vi "Write comments to sxp-file.vi"(5 "Location":enum16{"Beginning", "End"}(ring), 7 "Comment character":string="!", 8 "error in (no error)":errorcluster, 10 "Comment lines":string[](array[string]), 11 "file path":path) -> (0 "error out":errorcluster, 3 "file path out":path)   [LabVIEW 2020]
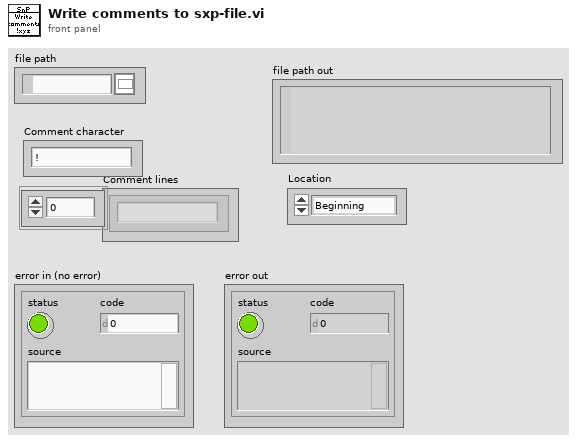
[diagram p1: front panel]
types:
  T1 = enum16{"open", "replace", "create", "open or create", "replace or create", "replace or create with confirmation"}
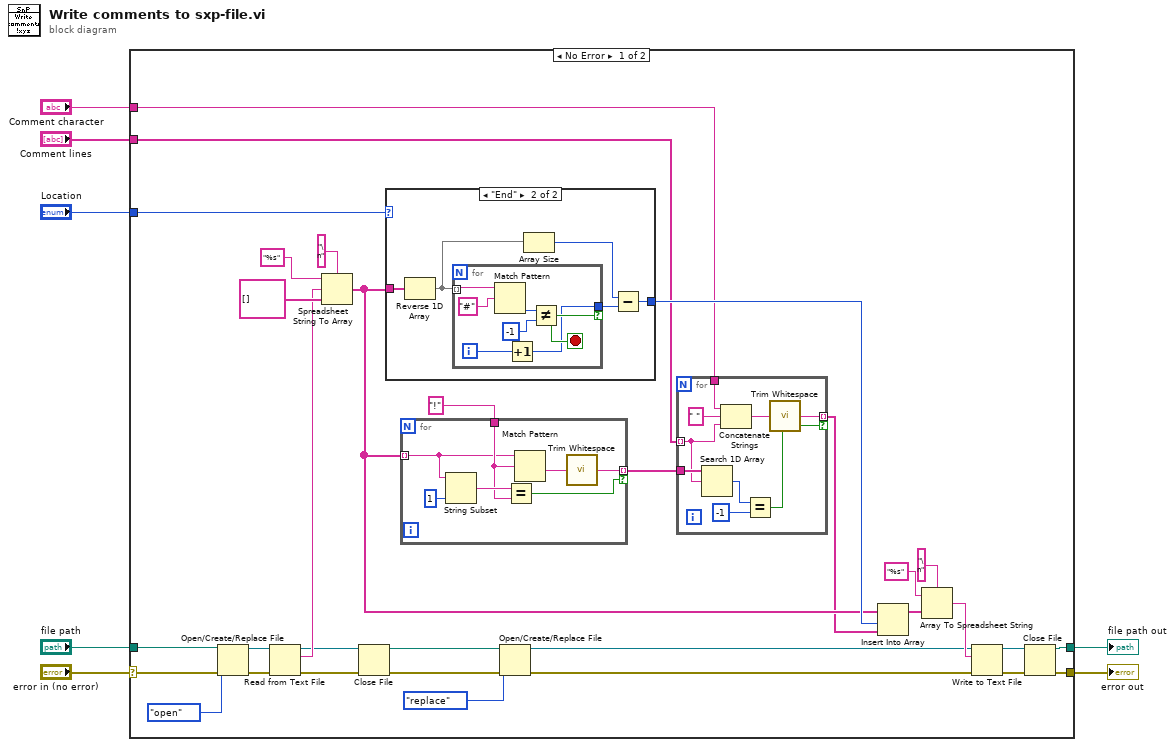
[diagram p0: block diagram]
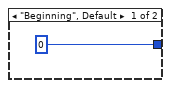
[diagram p2: hidden frame]
diagram:
  n1 = case shown="No Error" "error in (no error)" {
    selector: "error in (no error)" -> [w37 w70]
    tunnel: [w39 w70] -> w7
    tunnel: [w38 w69] -> w6
    tunnel: "Comment character" -> [w9 _]
    tunnel: "Comment lines" -> [w8 _]
    tunnel: "Location" -> [w24 _]
    tunnel: "file path" -> [w20 w69]
    frame No Error {
      n2 = Open/Create/Replace File(file path (use dialog)=w20, error in=w37, operation (0:open)=T1."open") -> (refnum out=w33:refnum<file>, error out=w32:errorcluster)  [unwired: 3 in, 1 out]
      n3 = Read from Text File(file (use dialog)=w33, error in=w32) -> (refnum out=w18:refnum<file>, text=w31:string, error out=w19:errorcluster)  [unwired: 2 in, 1 out]
      n4 = Spreadsheet String To Array(delimiter (Tab)="\n", format string="%s", spreadsheet string=w31, array type (2D Dbl)=string[] []) -> (array=w12:string[])
      n5 = Close File(refnum=w18, error in=w19) -> (path=w17:path, error out=w16:errorcluster)
      n6 = case shown="\"End\"" w24 {
        tunnel: [0 w57] -> w23
        tunnel: w12 -> [_ w58]
        frame "Beginning", Default {
        }
        frame "End" {
          n7 = Reverse 1D Array(array=w58) -> (reversed array=w59:string[])
          n8 = for {
            tunnel: w59 -> [w68] mode=indexing
            tunnel: [w62] -> w61 if=w64
            i -> [w63]
            stop <- w64 stop-if-true
            n9 = Match Pattern(string=w68, regular expression="#") -> (offset past match=w66:i32)  [unwired: 1 in, 3 out]
            n10 = Increment(x=w63) -> (x+1=w62:i32)
            n11 = Not Equal?(x=w66, y=-1) -> (x != y?=w64:bool)
          }
          n12 = Array Size(array=w59) -> (size(s)=w60:i32)
          n13 = Subtract(x=w60, y=w61) -> (x-y=w57:i32)
        }
      }
      n14 = for {
        tunnel: w12 -> [w51] mode=indexing
        tunnel: [w49] -> w11 mode=indexing if=w53
        tunnel: "!" ("Comment character 2") -> [w52]
        n15 = String Subset(string=w51, length (rest)=1 ("length (rest)")) -> (substring=w54:string)  [unwired: 1 in]
        n16 = Equal?(x=w54, y=w52) -> (x = y?=w53:bool)
        n17 = Match Pattern(string=w51, regular expression=w52) -> (after substring=w50:string)  [unwired: 1 in, 3 out]
        n18 = call <vilib>:"Trim Whitespace.vi"("string"=w50) -> ("trimmed string"=w49:string)  [unwired: 1 in]
      }
      n19 = Open/Create/Replace File(file path (use dialog)=w17, error in=w16, operation (0:open)=T1."replace") -> (refnum out=w15:refnum<file>, error out=w14:errorcluster)  [unwired: 3 in, 1 out]
      n20 = for {
        tunnel: w8 -> [w41] mode=indexing
        tunnel: w11 -> [w48]
        tunnel: [w40] -> w10 mode=indexing if=w45
        tunnel: w9 -> [w42]
        n21 = Search 1D Array(1D array=w48, element=w41) -> (index of element=w47:i32)  [unwired: 1 in]
        n22 = Concatenate Strings(w42, " " ("string"), w41) -> (w44:string)
        n23 = Equal?(x=w47, y=-1) -> (x = y?=w45:bool)
        n24 = call <vilib>:"Trim Whitespace.vi"("string"=w44) -> ("trimmed string"=w40:string)  [unwired: 1 in]
      }
      n25 = Insert Into Array(array=w12, index=w23, new element=w10) -> (w25:string[])
      n26 = Array To Spreadsheet String(delimiter (Tab)="\n", array=w25, 3:"%s" ("format string")) -> (spreadsheet string=w27:string)
      n27 = Write to Text File(file (use dialog)=w15, text=w27, error in=w14) -> (refnum out=w30:refnum<file>, error out=w29:errorcluster)  [unwired: 1 in, 1 out]
      n28 = Close File(refnum=w30, error in=w29) -> (path=w38:path, error out=w39:errorcluster)
    }
    frame Error {
    }
  }
  "error out" <- w7
  "file path out" <- w6
